vi "ReadSystemData.vi"(8 "error in (no error)":errorcluster) -> (0 "error out":errorcluster, 2 "SystemData Out":T1={"Message"={"UI"=refnum, "Task"=refnum, "Motor"=refnum, "DAQ"=refnum, "Logging"=refnum}, "ThisVIParameter"={"Stop"=refnum, "VI Path"=path "", "Data Path"=path "", "This VI Ref"=refnum, "UI Ctrls"={"Menu"=refnum, "Start"=refnum, "Stop"=refnum, "Home"=refnum, "Virtual"=refnum, "Save"=refnum}}, "DBLink"="", "DeployProject"="", "Project.lvclass"=refnum, "StepDataArray"=[], "RuntimeIdx"=0, "HomeIdx"=0, "DAQ Hardware"={"Task"="", "Max"=5.0, "min"=-5.0, "Samples Rate"=1000.0, "Channels"=[]}, "Serial Settings"={"VISA"="", "Baud Rate"=9600, "Data Bits"=8, "Parity"=enum."None", "Stop Bits"=10, "Flow Control"=0}, "Display"={"DataArray"=refnum, "X"=refnum, "Y"=refnum, "Z"=refnum, "R"=refnum, "Data"=refnum}, "Streaming"={"Datas"=refnum, "Ready X"=0.0, "Ready Y"=0.0, "Ready Z"=0.0, "Ready R"=0.0, "DataArray"=[]}, "Read"={"Sensor No."=0, "Log?"=FALSE}, "VirtualDataArray"=[], "VirtualIdx"=0, "VirtualXIdx"=0, "VirtualYIdx"=0, "VirtualXArray"=[], "VirtualYArray"=[], "Mode"=enum."Auto", "Standby"=[], "StandbyIdx"=0} {"Serial Settings"."Flow Control" items=["None"=0, "XON/XOFF"=1, "RTS/CTS"=2, "DTR/DSR"=4]; "Serial Settings"."Stop Bits" items=["1.0"=10, "1.5"=15, "2.0"=20]; "Serial Settings"."Data Bits" min=5 max=8 step=1; "Serial Settings"."Baud Rate" items=["75"=75, "110"=110, "134"=134, "150"=150, "300"=300, "600"=600, "1200"=1200, "1800"=1800, "2400"=2400, "4800"=4800, "7200"=7200, "9600"=9600, "14400"=14400, "19200"=19200, "28800"=28800, "38400"=38400, "56000"=56000, "57600"=57600, "115200"=115200, "128000"=128000, "230400"=230400]; "DAQ Hardware"."min" format="%0.2f"; "DAQ Hardware"."Max" format="%0.2f"})   [LabVIEW 2014, in "SystemData.lvclass"]
uses:
  SystemData.lvclass
  SystemDataTypeDefine.ctl
  ProjectAndStep/Project/Project.lvclass
  Message Queue/All Message Queues.ctl
  Message Queue/Message Cluster.ctl
  Controls/UI Controls.ctl
  ProjectAndStep/StepData/StepData.lvclass
  NIDAQ/DAQHardware.ctl
  Display Notifier/All Display Notifiers.ctl
  Controls/Streaming.ctl
  ProjectAndStep/StepData/Control/MeasureData.ctl
  ProjectAndStep/Virtual/VirtualOrigin.lvclass
  Controls/Mode Controls.ctl
  Singleton.lvclass/Singleton.lvclass/Singleton.ctl
  SystemData.lvclass/SystemData.ctl
  Singleton.lvclass/Constructor.vi
  Singleton.lvclass/Singleton.lvclass
  Message Queue/Message Queue.lvlib
  NIDAQ/NIDAQ.lvlib
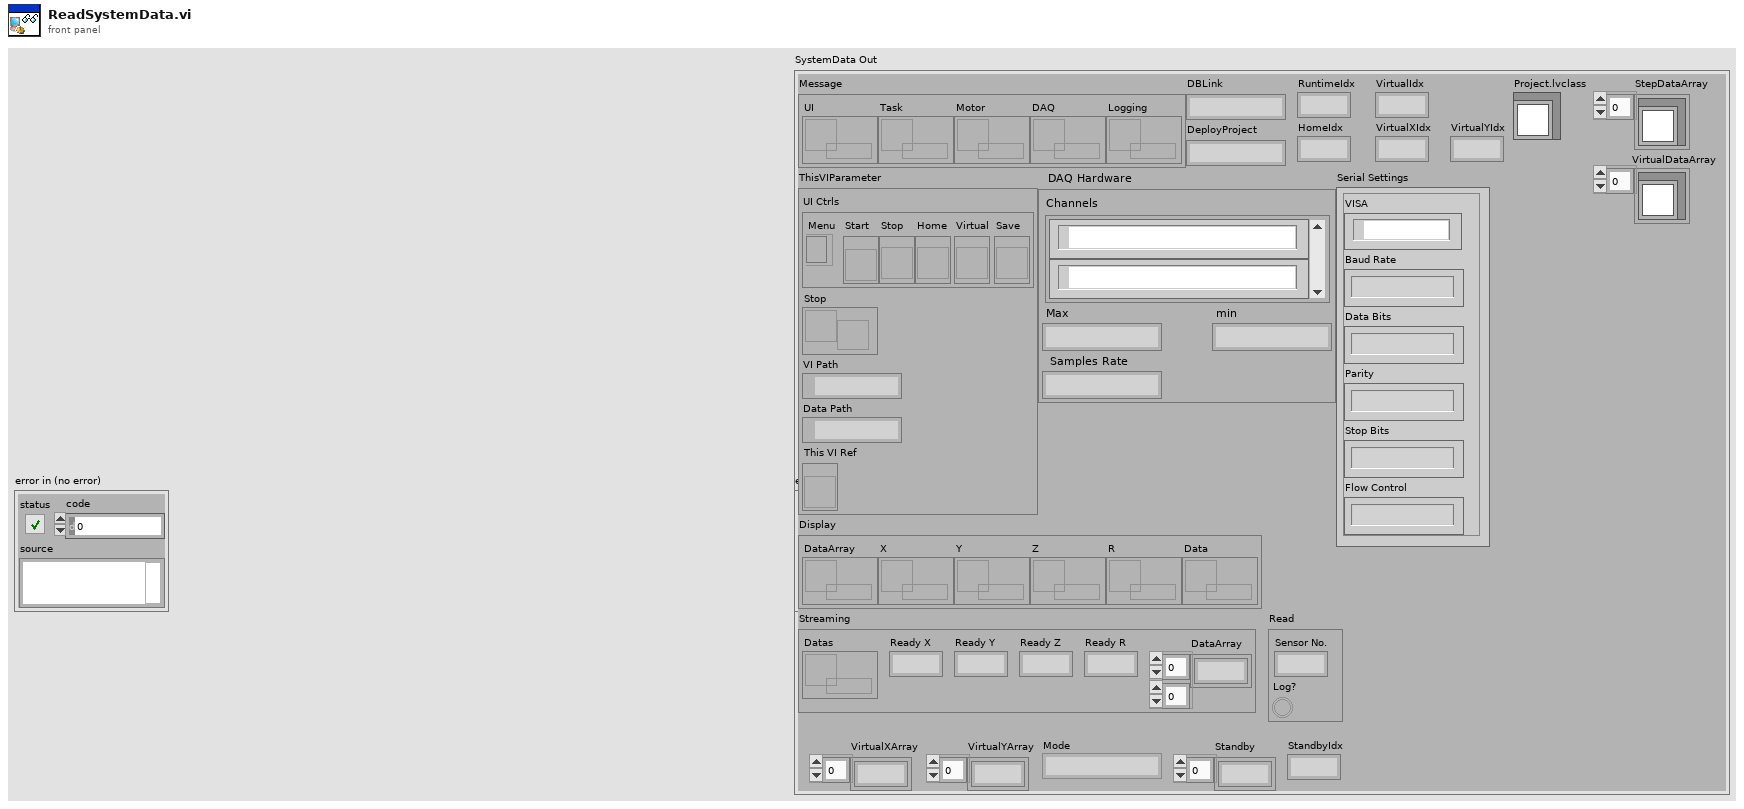
[diagram p1: front panel]
types:
  T1 = typedef "SystemData.lvclass/SystemDataTypeDefine.ctl" = cluster{"Message":T2, "ThisVIParameter":cluster{"Stop":refnum<user-event>, "VI Path":path, "Data Path":path, "This VI Ref":refnum<vi>, "UI Ctrls":T3}, "DBLink":string, "DeployProject":string, "Project.lvclass":refnum<class "Project.lvclass">, "StepDataArray":refnum<class "StepData.lvclass">[], "RuntimeIdx":i32, "HomeIdx":i32, "DAQ Hardware":T4, "Serial Settings":cluster{"VISA":refnum<visa-resource-name>, "Baud Rate":u32, "Data Bits":u16, "Parity":enum16{"None", "Odd", "Even", "Mark", "Space"}, "Stop Bits":u16, "Flow Control":u16}, "Display":T5, "Streaming":T6, "Read":T7, "VirtualDataArray":refnum<class "VirtualOrigin.lvclass">[], "VirtualIdx":i32, "VirtualXIdx":i32, "VirtualYIdx":i32, "VirtualXArray":dbl[], "VirtualYArray":dbl[], "Mode":T8, "Standby":dbl[], "StandbyIdx":i32}
  T2 = typedef "Message Queue.lvlib/All Message Queues.ctl" = cluster{"UI":refnum<queue>, "Task":refnum<queue>, "Motor":refnum<queue>, "DAQ":refnum<queue>, "Logging":refnum<queue>}
  T3 = typedef "UI Controls.ctl" = cluster{"Menu":refnum<k9>, "Start":refnum<vi>, "Stop":refnum<vi>, "Home":refnum<vi>, "Virtual":refnum<vi>, "Save":refnum<vi>}
  T4 = typedef "NIDAQ.lvlib/DAQHardware.ctl" = cluster{"Task":refnum<k21>, "Max":dbl, "min":dbl, "Samples Rate":dbl, "Channels":tag[]}
  T5 = typedef "All Display Notifiers.ctl" = cluster{"DataArray":refnum<queue>, "X":refnum<queue>, "Y":refnum<queue>, "Z":refnum<queue>, "R":refnum<queue>, "Data":refnum<queue>}
  T6 = typedef "Streaming.ctl" = cluster{"Datas":refnum<queue>, "Ready X":dbl, "Ready Y":dbl, "Ready Z":dbl, "Ready R":dbl, "DataArray":dbl[][]}
  T7 = typedef "StepData.lvclass/MeasureData.ctl" = cluster{"Sensor No.":i32, "Log?":bool}
  T8 = typedef "Mode Controls.ctl" = enum16{"Auto", "Virtual", "Home", "Standby"}
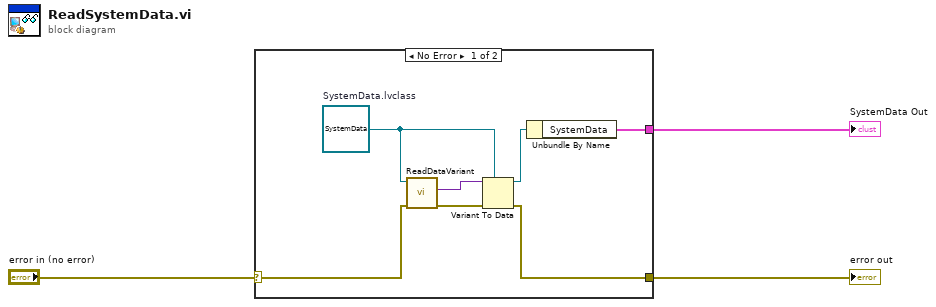
[diagram p0: block diagram]
diagram:
  n1 = case shown="No Error" "error in (no error)" {
    selector: "error in (no error)" -> [w6 w11]
    tunnel: [w4 w11] -> w2
    tunnel: [w7 _] -> w1
    frame No Error {
      w9 = refnum<class "SystemData.lvclass"> refnum  # SystemData.lvclass
      n2 = call "ReadDataVariant.vi"("error in (no error)"=w6, "Singleton.lvclass In"=w9) -> ("error out"=w5:errorcluster, "DataVariant"=w10:variant)  [unwired: 7 in, 1 out]
      n3 = Variant To Data(error in=w5, type=w9, Variant=w10) -> (data=w8:refnum<class "SystemData.lvclass">, error out=w4:errorcluster)
      n4 = Unbundle By Name(w8) -> ("SystemData"=w7:T1)
    }
    frame Error {
    }
  }
  "error out" <- w2
  "SystemData Out" <- w1
